vi "HandleVersionMutation.vi"(4 "To Version":u16, 6 "From Version":u16, 8 "error in (no error)":errorcluster, 10 "SerializableData in":variant, 11 "Hulk Hogan":refnum<class "Hulk Hogan.lvclass">) -> (0 "error out":errorcluster, 2 "SerializableData out":variant, 3 "Hulk Hogan":refnum<class "Hulk Hogan.lvclass">)   [LabVIEW 2020, in "Hulk Hogan.lvclass"]
uses:
  Hulk Hogan.lvclass
  SerializableData_v1.ctl
  SerializableData_v2.ctl
  <vilib>/Utility/error.llb/Error Cluster From Error Code.vi
  <vilib>/ErrorRing/Error Ring.xnode
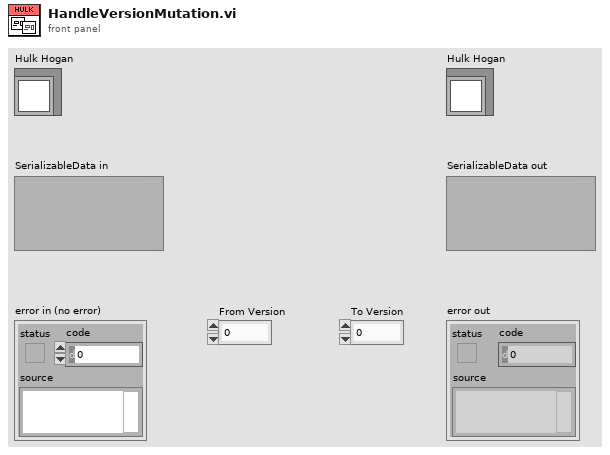
[diagram p1: front panel]
types:
  T1 = typedef "Hulk Hogan.lvclass/SerializableData_v1.ctl" = cluster{"HulkNumber":dbl}
  T2 = typedef "Hulk Hogan.lvclass/SerializableData_v2.ctl" = cluster{"HulkNumber":string}
  T3 = typedef "Hulk Hogan.lvclass/SerializableData.ctl" = cluster{"HulkNumber":enum16{"e", "pi", "c"}}
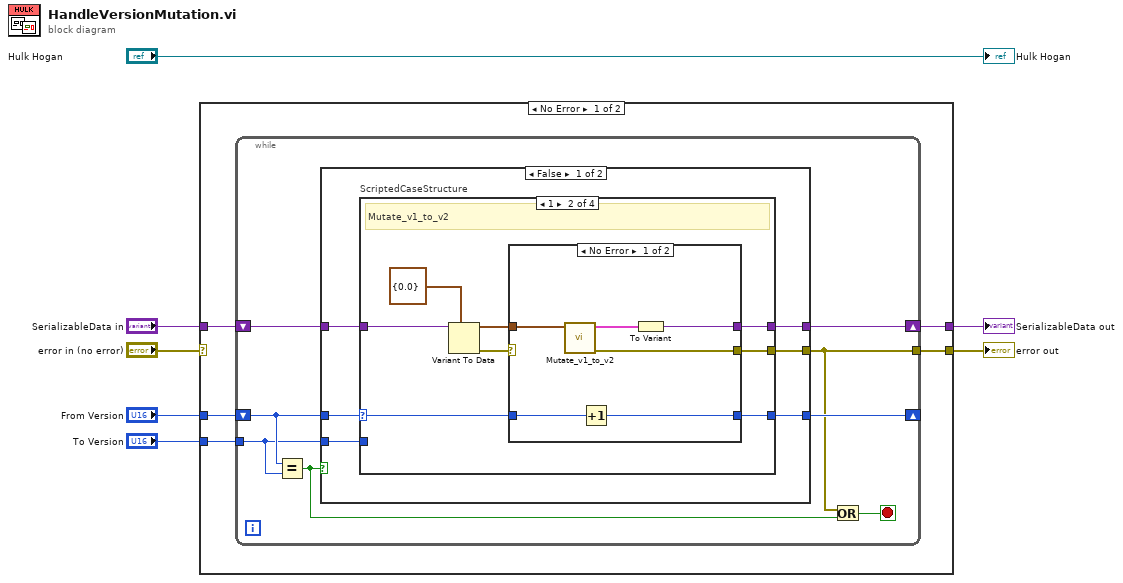
[diagram p0: block diagram]
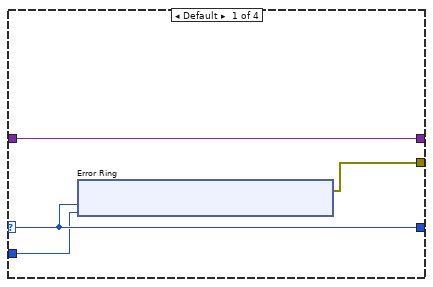
[diagram p2: hidden frame]
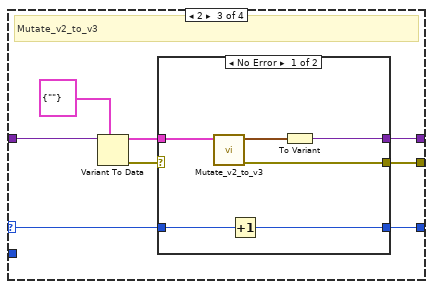
[diagram p4: hidden frame]
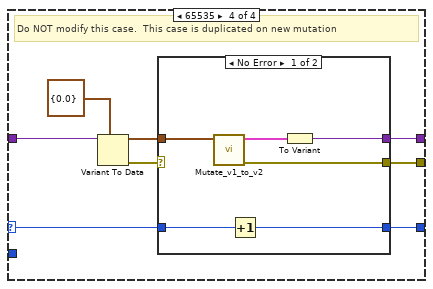
[diagram p6: hidden frame]
diagram:
  n1 = case shown="No Error" "error in (no error)" {
    selector: "error in (no error)" -> [_ w90]
    tunnel: "From Version" -> [w12 _]
    tunnel: "To Version" -> [w11 _]
    tunnel: "SerializableData in" -> [w10 w89]
    tunnel: [w9 w90] -> w4
    tunnel: [w8 w89] -> w3
    frame No Error {
      n2 = while {
        tunnel: w11 -> [w13]
        shift-right: [w17] -> _
        shift-left: w12 -> [w20]
        shift-right: [w18] -> w8
        shift-left: w10 -> [w19]
        tunnel: [w14] -> w9
        stop <- w15 stop-if-true
        n3 = Equal?(x=w20, y=w13) -> (x = y?=w16:bool)
        n4 = case shown="False" w16 {
          tunnel: w20 -> [w26 w88]
          tunnel: w19 -> [w25 w87]
          tunnel: [w24 w87] -> w18
          tunnel: [w23 _] -> w14
          tunnel: [w22 w88] -> w17
          tunnel: w13 -> [w21 _]
          frame False {
            n5 = case "ScriptedCaseStructure" shown="1" w26 {
              selector: w26 -> [w30 w40 w56 w72]
              tunnel: w25 -> [w28 w46 w62 w78]
              tunnel: [w28 w43 w59 w75] -> w24
              tunnel: [w29 w42 w58 w74] -> w23
              tunnel: [w30 w41 w57 w73] -> w22
              tunnel: w21 -> [w27 _ _ _]
              frame Default {
                n6 = xnode "Error Ring"("parameter 0"=w30, "parameter 1"=w27) -> ("error out"=w29:errorcluster)
              }
              frame 1 {
                # "Mutate_v1_to_v2"
                n7 = Variant To Data(type=T1 {"HulkNumber"=0.0} ("SerializableData"), Variant=w46) -> (data=w44:T1, error out=w45:errorcluster)  [unwired: 1 in]
                n8 = case shown="No Error" w45 {
                  selector: w45 -> [_ w54]
                  tunnel: w44 -> [w49 _]
                  tunnel: [w52 _] -> w43
                  tunnel: [w47 w54] -> w42
                  tunnel: w40 -> [w51 w53]
                  tunnel: [w50 w53] -> w41
                  frame No Error {
                    n9 = call "Mutate_v1_to_v2.vi"("SerializableData_v1"=w49) -> ("error out"=w47:errorcluster, "SerializableData_v2"=w48:T2)  [unwired: 9 in]
                    n10 = Increment(x=w51) -> (x+1=w50:u16)
                    n11 = To Variant(anything=w48) -> (Variant=w52:variant)
                  }
                  frame Error {
                  }
                }
              }
              frame 2 {
                # "Mutate_v2_to_v3"
                n12 = Variant To Data(type=T2 {"HulkNumber"=""} ("SerializableData"), Variant=w62) -> (data=w60:T2, error out=w61:errorcluster)  [unwired: 1 in]
                n13 = case shown="No Error" w61 {
                  selector: w61 -> [_ w70]
                  tunnel: w60 -> [w65 _]
                  tunnel: [w68 _] -> w59
                  tunnel: [w63 w70] -> w58
                  tunnel: w56 -> [w67 w69]
                  tunnel: [w66 w69] -> w57
                  frame No Error {
                    n14 = call "Mutate_v2_to_v3.vi"("SerializableData_v2"=w65) -> ("error out"=w63:errorcluster, "SerializableData"=w64:T3)  [unwired: 9 in]
                    n15 = Increment(x=w67) -> (x+1=w66:u16)
                    n16 = To Variant(anything=w64) -> (Variant=w68:variant)
                  }
                  frame Error {
                  }
                }
              }
              frame 65535 {
                # "Do NOT modify this case.  This case is duplicated on new mutation"
                n17 = Variant To Data(type=T1 {"HulkNumber"=0.0} ("SerializableData"), Variant=w78) -> (data=w76:T1, error out=w77:errorcluster)  [unwired: 1 in]
                n18 = case shown="No Error" w77 {
                  selector: w77 -> [_ w86]
                  tunnel: w76 -> [w81 _]
                  tunnel: [w84 _] -> w75
                  tunnel: [w79 w86] -> w74
                  tunnel: w72 -> [w83 w85]
                  tunnel: [w82 w85] -> w73
                  frame No Error {
                    n19 = call "Mutate_v1_to_v2.vi"("SerializableData_v1"=w81) -> ("error out"=w79:errorcluster, "SerializableData_v2"=w80:T2)  [unwired: 9 in]
                    n20 = Increment(x=w83) -> (x+1=w82:u16)
                    n21 = To Variant(anything=w80) -> (Variant=w84:variant)
                  }
                  frame Error {
                  }
                }
              }
            }
          }
          frame True {
          }
        }
        n22 = Or(x=w14, y=w16) -> (x .or. y?=w15:bool)
      }
    }
    frame Error {
    }
  }
  "error out" <- w4
  "SerializableData out" <- w3
  "Hulk Hogan" <- "Hulk Hogan"
